vi "ex7-2.vi"   [LabVIEW 2013]
uses:
  <vilib>/NXT/Block Support/NXT_InputPort.ctl
  <vilib>/NXT/Dual Mode Library/Sensors/EV3_Color_Reflect.vi
  <vilib>/NXT/Dual Mode Library/prims/inRangeAndCoerce/inRangeAndCoerce_float.vi
  <vilib>/NXT/Dual Mode Library/Display/drawNumber.vi
types:
  T1 = typedef "NXT_InputPort.ctl" = u32
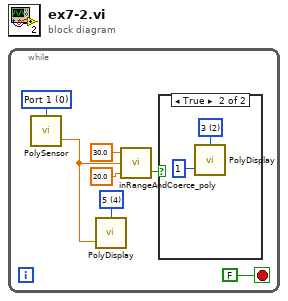
[diagram p0: block diagram]
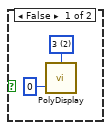
[diagram p2: hidden frame]
diagram:
  n1 = while {
    stop <- FALSE stop-if-true
    w2 = i16 4 items=["1", "2", "3", "4", "5", "6", "7", "8", "9", "10", "11", "12"] ("Line")
    w6 = T1 0 items=["Port 1", "Port 2", "Port 3", "Port 4"] ("Port (Port 3)")
    n2 = call-poly <vilib>:"PolySensor.vi"("Port (Port 1)"=w6) -> ("Scaled Value"=w1:sgl)  [unwired: 2 in, 1 out]
    n3 = call-poly <vilib>:"PolyDisplay.vi"("number"=w1, "Line"=w2) -> ()  [unwired: 2 in, 1 out]
    n4 = call-poly <vilib>:"inRangeAndCoerce_poly.vi"("lower limit"=sgl 20.0, "x"=w1, "upper limit"=sgl 30.0) -> ("In Range?"=w5:bool)  [unwired: 1 out]
    n5 = case shown="True" w5 {
      frame False {
        w9 = i16 2 items=["1", "2", "3", "4", "5", "6", "7", "8", "9", "10", "11", "12"] ("Line")
        n6 = call-poly <vilib>:"PolyDisplay.vi"("number"=0, "Line"=w9) -> ()  [unwired: 2 in, 1 out]
      }
      frame True {
        w11 = i16 2 items=["1", "2", "3", "4", "5", "6", "7", "8", "9", "10", "11", "12"] ("Line")
        n7 = call-poly <vilib>:"PolyDisplay.vi"("number"=1, "Line"=w11) -> ()  [unwired: 2 in, 1 out]
      }
    }
  }
